vi "Get Selected Aircraft.vi"(8 "Error In":errorcluster) -> (0 "Error Out":errorcluster, 3 "Selected Aircraft ID Out":u8)   [LabVIEW 2014]
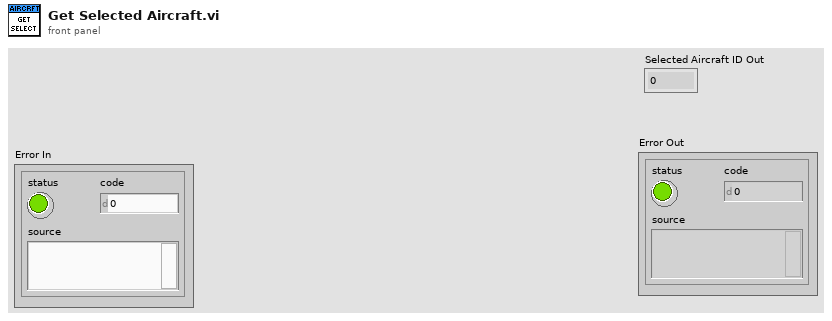
[diagram p1: front panel]
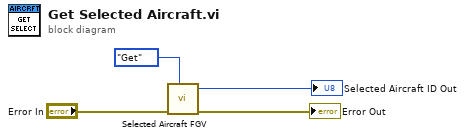
[diagram p0: block diagram]
diagram:
  n1 = call "Selected Aircraft FGV.vi"("Operation"=enum16{"Get", "Set"}."Get", "Error In"="Error In") -> ("Error Out"=→"Error Out":errorcluster, "Selected Aircraft ID Out"=→"Selected Aircraft ID Out":u8)  [unwired: 8 in]
